vi "GV stage pulse stretcher.vi"() -> ()   [LabVIEW 2017]
panel:
  out "StagePulseStretcher_tick":u32
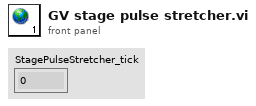
[diagram p1: front panel]
diagram:
